vi "Set separate code.vi"() -> ()   [LabVIEW 2015]
panel:
  in  "Stop on bad":bool=TRUE
  out "Execution:State":T1(ring)
  out "Modified files":path[](array[path])
  out "Modified":i32
  in  "Stop Button":bool
  out "File Path":path
  out "Progress":string
  in  "Folder Path":path
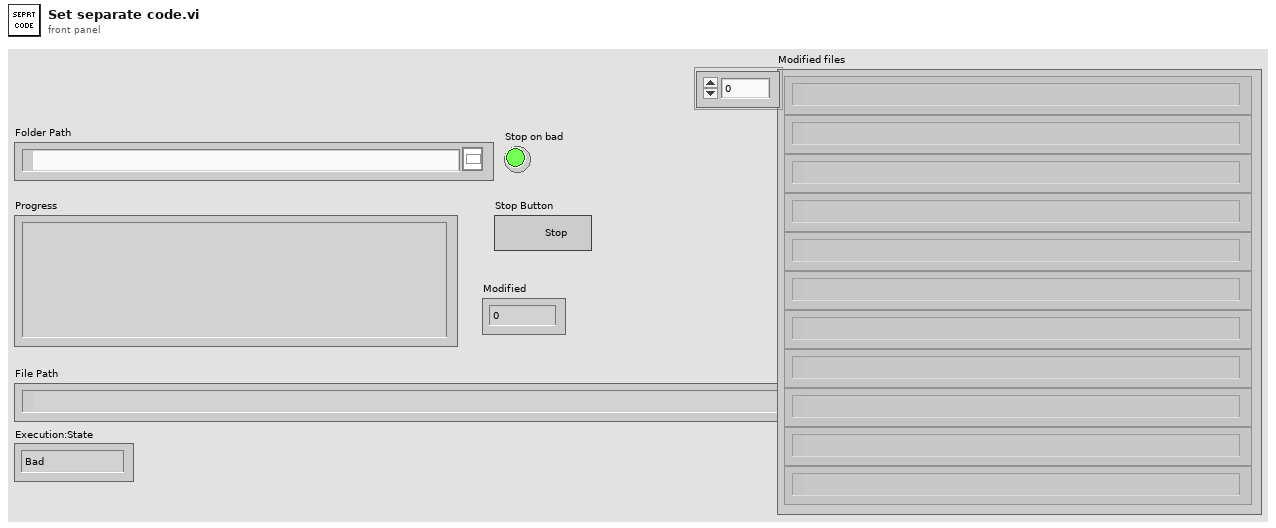
[diagram p1: front panel]
types:
  T1 = enum32{"Bad", "Idle", "Run top level", "Running"}
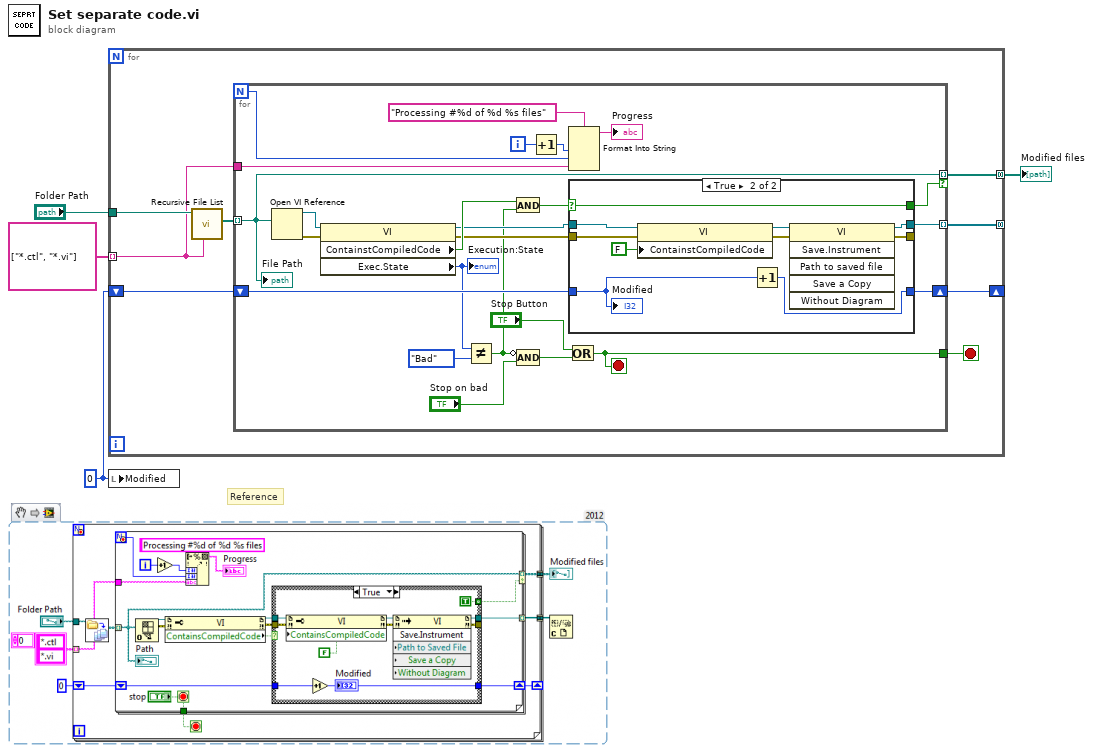
[diagram p0: block diagram]
diagram:
  w1 = 0 ("Modified")
  # "Reference"
  n1 = for {
    tunnel: string[] ["*.ctl", "*.vi"] -> [w10] mode=indexing
    shift-right: [w7] -> _
    shift-left: w1 -> [w8]
    tunnel: "Folder Path" -> [w12]
    tunnel: [w6] -> _ mode=concatenating
    tunnel: [w5] -> w2 mode=concatenating
    stop <- w9 stop-if-true
    n2 = call <vilib>:"Recursive File List.vi"("pattern"=w10, "Folder Path"=w12) -> ("All Files in Dir"=w11:path[])  [unwired: 5 in, 4 out]
    n3 = for {
      N -> [w33]
      tunnel: w11 -> [w21] mode=indexing
      tunnel: w10 -> [w32]
      tunnel: [w14] -> w9
      tunnel: [w24] -> w6 mode=indexing
      shift-right: [w22] -> w7
      shift-left: w8 -> [w23]
      tunnel: [w21] -> w5 mode=indexing if=w20
      i -> [w35]
      stop <- w14 stop-if-true
      n4 = Open VI Reference(vi path=w21) -> (vi reference=w30:refnum<vi>, error out=w29:errorcluster)  [unwired: 5 in]
      n5 = property class="VI"(reference=w30, error in=w29) -> (reference out=w26:refnum<vi>, error out=w25:errorcluster, "ContainstCompiledCode"=w27:bool, "Exec.State"=w19:T1)
      "Execution:State" <- w19
      n6 = Not Equal?(x=w19, y=T1."Bad" ("Execution:State")) -> (x != y?=w16:bool)
      n7 = And(x=w27, y=w16) -> (x .and. y?=w17:bool)
      n8 = Compound Arithmetic op=AND(invert w16, "Stop on bad") -> (w13:bool)
      n9 = Increment(x=w35) -> (x+1=w34:i32)
      n10 = Or(x="Stop Button", y=w13) -> (x .or. y?=w14:bool)
      n11 = Format Into String(format string="Processing #%d of %d %s files", w34, w33, w32) -> (resulting string=→"Progress":string)  [unwired: 2 in, 1 out]
      n12 = case shown="True" w17 {
        selector: w17 -> [w37 w42]
        tunnel: w26 -> [w39 w49]
        tunnel: w25 -> [w40 w48]
        tunnel: [w40 w45] -> _
        tunnel: [w39 w44] -> w24
        tunnel: w23 -> [w38 w41]
        tunnel: [w38 w43] -> w22
        tunnel: [w37 w42] -> w20
        frame False {
        }
        frame True {
          n13 = property class="VI"(reference=w49, error in=w48, "ContainstCompiledCode"=FALSE ("Contains Compiled Code")) -> (reference out=w47:refnum<vi>, error out=w46:errorcluster)
          n14 = Increment(x=w41) -> (x+1=w43:i32)
          n15 = invoke class="VI" method="Save.Instrument"(reference=w47, error in=w46) -> (reference out=w44:refnum<vi>, error out=w45:errorcluster)  [unwired: 4 in, 4 out]
          "Modified" <- w41
        }
      }
      "File Path" <- w21
    }
  }
  "Modified files" <- w2
  n16 = local write "Modified"(w1) -> ()
